vi "MODBUS_NANODAC.vi"() -> (0 "error out":errorcluster, 3 "Modbus Master out":refnum<class "Modbus Master.lvclass">, 5 "Status CO":bool, 6 "Status LEL":bool, 7 "Status O2":bool, 9 "LEL (%)":dbl, 10 "CO (ppm)":dbl, 11 "O2 (%)":dbl)   [LabVIEW 2021, in "CC_Library.lvlib"]
uses:
  CC_Library.lvlib
  <vilib>/Modbus/master/Modbus Master.lvclass
  <vilib>/Modbus/master/Create Master Instance (TCP).vi
panel:
  in  "Stop ALL":refnum<vi>
  out "Loop Rate (Hz) Electro 2":dbl format="%#_2g"
  out "H2,O2,CO":dbl[](array[numeric])
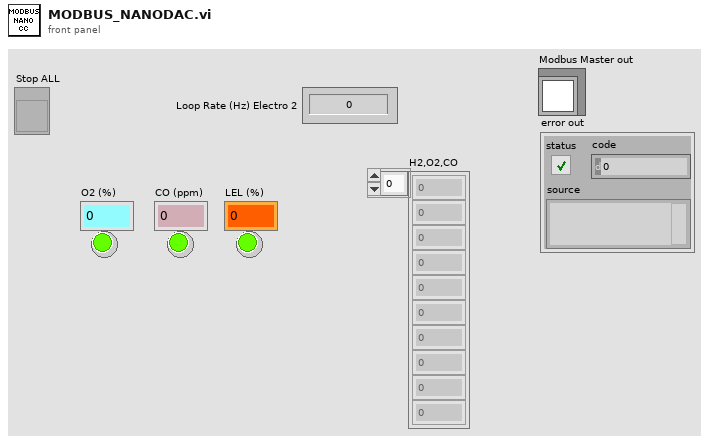
[diagram p1: front panel]
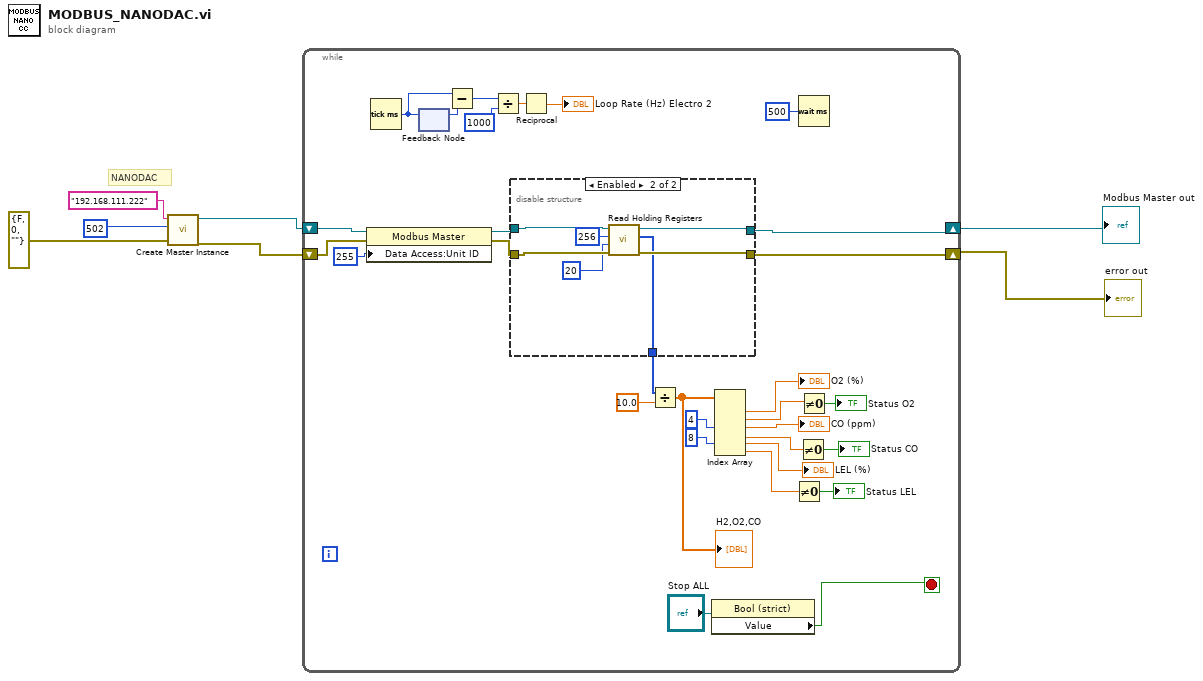
[diagram p0: block diagram]
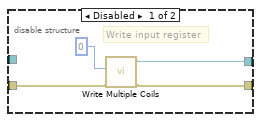
[diagram p2: hidden frame]
diagram:
  # "NANODAC"
  n1 = call-poly <vilib>:"Create Master Instance.vi"("error in (no error)"=errorcluster {"status"=FALSE, "code"=0, "source"=""}, "port (502)"=u16 502, "address"="192.168.111.222") -> ("error out"=w3:errorcluster, "TCP master instance"=w4:refnum<class "Modbus Master.lvclass">)  [unwired: 7 in]
  n2 = while {
    shift-right: [w29] -> w2
    shift-left: w4 -> [w28]
    shift-right: [w30] -> w1
    shift-left: w3 -> [w27]
    stop <- w8 stop-if-true
    n3 = property class="Modbus Master"(reference=w28, error in=w27, "Data Access:Unit ID"=u8 255 ("Unit ID")) -> (reference out=w26:refnum<class "Modbus Master.lvclass">, error out=w25:errorcluster)
    n4 = Tick Count (ms)() -> (millisecond timer value=w36:u32)
    n5 = feedback #1() -> (w37:u32)  [unwired: 1 in]
    n6 = feedback-in #1(w36) -> ()
    n7 = Subtract(x=w36, y=w37) -> (x-y=w35:u32)
    n8 = Divide(x=w35, y=u32 1000) -> (x/y=w33:dbl)
    n9 = disable-structure shown="Enabled" {
      disable-tunnel: [w43 w49] -> w29
      disable-tunnel: [w40 w48] -> w30
      disable-tunnel: w25 -> [w38 w47]
      disable-tunnel: w26 -> [_ w45]
      disable-tunnel: [_ w44] -> w22
      frame Disabled {
        # "Write input register"
        n10 = call-dynamic "Write Multiple Coils.vi"("error in (no error)"=w38, "starting address"=u16 0) -> ("error out"=w40:errorcluster, "Modbus master out"=w43:refnum<class "Modbus Master.lvclass">, "coil values"=w41:bool[], "Modbus master in"=w39:refnum<class "Modbus Master.lvclass">)  [unwired: 6 in]
      }
      frame Enabled {
        n11 = call-dynamic "Read Holding Registers.vi"("error in (no error)"=w47, "number of holding registers"=u16 20, "starting address"=u16 256 ("address"), "Modbus master in"=w45) -> ("error out"=w48:errorcluster, "register values"=w44:u16[], "Modbus master out"=w49:refnum<class "Modbus Master.lvclass">)  [unwired: 5 in]
      }
    }
    n12 = Reciprocal(x=w33) -> (1/x=→"Loop Rate (Hz) Electro 2":dbl)
    n13 = Divide(x=w22, y=10.0) -> (x/y=w21:dbl[])
    "H2,O2,CO" <- w21
    n14 = property class="Bool (strict)"(reference="Stop ALL") -> ("Value"=w8:bool)  [unwired: 1 in, 2 out]
    n15 = Index Array(array=w21, index #3=4 ("index"), index #5=8 ("index")) -> (element #1=→"O2 (%)":dbl, element #2=w13:dbl, element #3=→"CO (ppm)":dbl, element #4=w15:dbl, element #5=→"LEL (%)":dbl, element #6=w14:dbl)  [unwired: 4 in]
    n16 = Not Equal To 0?(x=w14) -> (x != 0?=→"Status LEL":bool)
    n17 = Not Equal To 0?(x=w15) -> (x != 0?=→"Status CO":bool)
    n18 = Wait (ms)(milliseconds to wait=u32 500) -> ()  [unwired: 1 out]
    n19 = Not Equal To 0?(x=w13) -> (x != 0?=→"Status O2":bool)
  }
  "Modbus Master out" <- w2
  "error out" <- w1
